vi "file_io_1.vi"() -> ()   [LabVIEW 2017]
uses:
  <vilib>/Utility/file.llb/Read Delimited Spreadsheet (string).vi
panel:
  out "EOF?":bool
  out "all rows":string[][](array[string])
  out "text":string
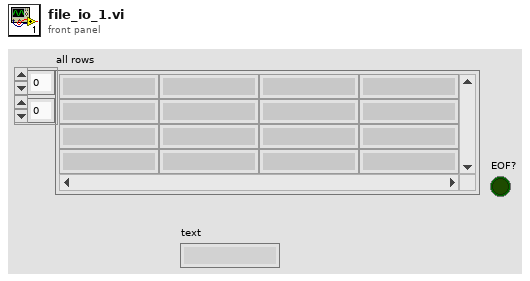
[diagram p1: front panel]
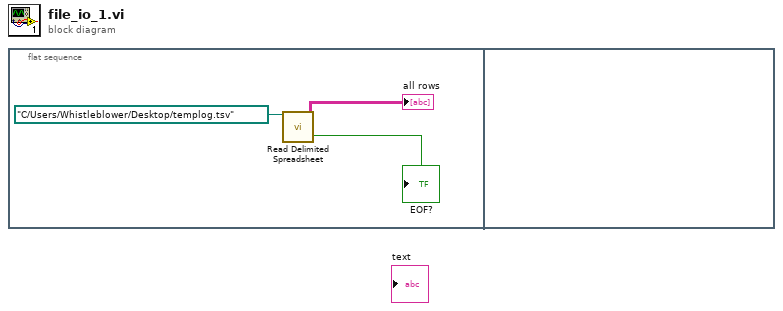
[diagram p0: block diagram]
diagram:
  n1 = flat-sequence {
    frame #0 {
      n2 = call-poly <vilib>:"Read Delimited Spreadsheet.vi"("file path (dialog if empty)"=path "C:/Users/Whistleblower/Desktop/templog.tsv") -> ("all rows"=→"all rows":string[][], "EOF?"=→"EOF?":bool)  [unwired: 9 in, 4 out]
    }
    frame #1 {
    }
  }
